vi "GetRandomNum.vi"(8 "error in (no error)":errorcluster, 11 "Generator in":refnum<class "Generator.lvclass">) -> (0 "error out":errorcluster, 3 "Generator out":refnum<class "Generator.lvclass">)   [LabVIEW 2014, in "Generator.lvlib" / "Generator.lvclass"]
uses:
  Generator.lvclass
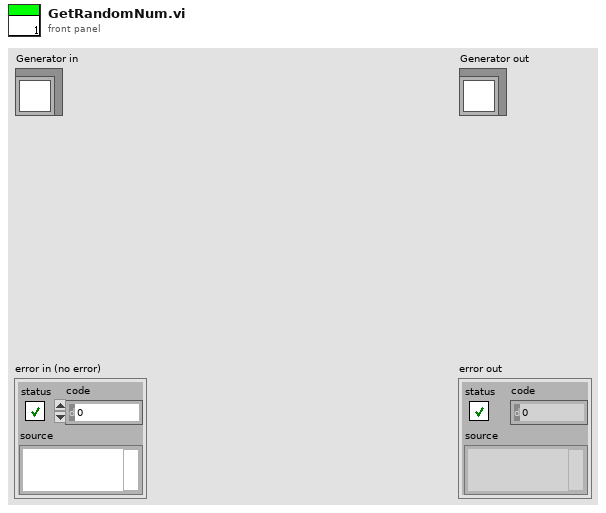
[diagram p1: front panel]
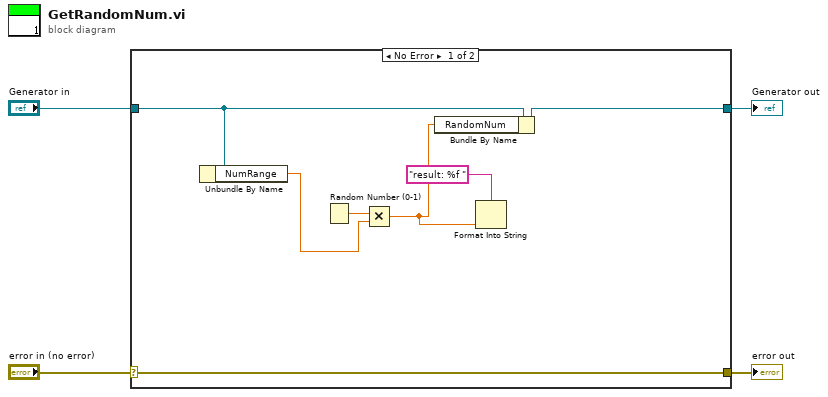
[diagram p0: block diagram]
diagram:
  n1 = case shown="No Error" "error in (no error)" {
    selector: "error in (no error)" -> [w11 w13]
    tunnel: [w11 w13] -> w3
    tunnel: [w9 w12] -> w1
    tunnel: "Generator in" -> [w6 w12]
    frame No Error {
      n2 = Unbundle By Name(w6) -> ("NumRange"=w5:dbl)
      n3 = Random Number (0-1)() -> (number: 0 to 1=w10:dbl)
      n4 = Multiply(x=w10, y=w5) -> (x*y=w7:dbl)
      n5 = Bundle By Name(cluster=w6, "RandomNum"=w7) -> (w9:refnum<class "Generator.lvclass">)
      n6 = Format Into String(format string="result: %f ", w7) -> ()  [unwired: 2 in, 2 out]
    }
    frame Error {
    }
  }
  "error out" <- w3
  "Generator out" <- w1
